vi "wykresy.vi"(8 "error in (no error)":errorcluster, 10 "x*y":dbl[](array[numeric]), 11 "wyjœcie":T1={"Runer's Data"={"Name"="", "Age"=0}, "HR Max"=0, "Raw Data"={"Time"=[], "Bpm"=[]}, "% HR MAX "=[], "HR Zones "=[], "no of points"=[], "Heart Rate Zone No 2"=[], "History"=[["training number", "HR Max value", "HR Mean value"], ["", "", ""]], "number history"=0}) -> (0 "error in (no error) 2":errorcluster, 3 "wyjœcie 2":T1={"Runer's Data"={"Name"="", "Age"=0}, "HR Max"=0, "Raw Data"={"Time"=[], "Bpm"=[]}, "% HR MAX "=[], "HR Zones "=[], "no of points"=[], "Heart Rate Zone No 2"=[], "History"=[["training number", "HR Max value", "HR Mean value"], ["", "", ""]], "number history"=0})   [LabVIEW 2024]
uses:
  zad_3-labview/klaster 4.ctl
  zad_3-labview/klaster.ctl
  zad_3-labview/klaster 2.ctl
panel:
  out "String 2":string
  out "String":string
  out "BPM":cluster{"Time":timestamp[], "Bpm":i32[]}(graph)
  in  "File Path":path
  in  "Button":bool
  out "HEART RATE ZONES":string[][](array[string])
  out "XY Graph":T4(graph)
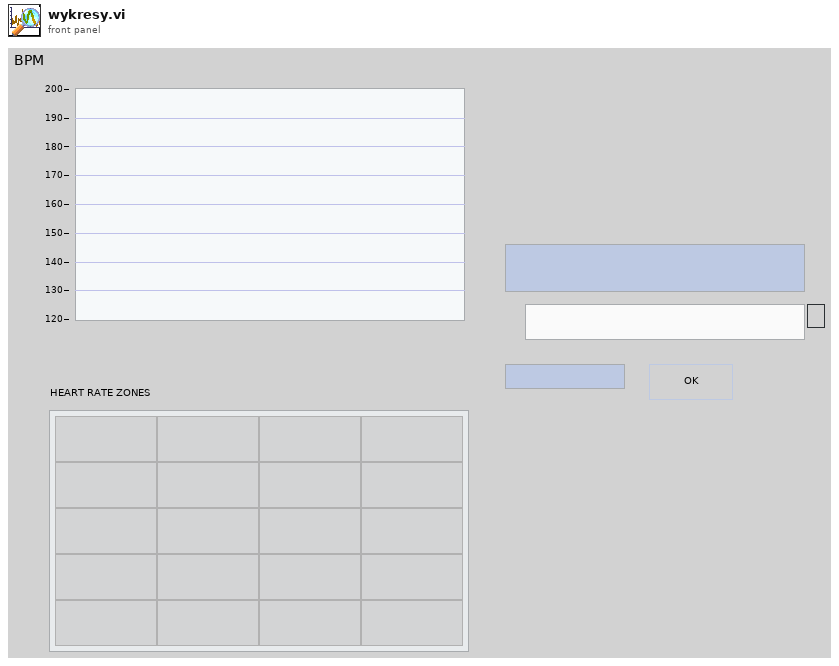
[diagram p1: front panel]
types:
  T1 = typedef "klaster 4.ctl" = cluster{"Runer's Data":T2, "HR Max":i32, "Raw Data":T3, "% HR MAX ":dbl[], "HR Zones ":string[][], "no of points":dbl[], "Heart Rate Zone No 2":i32[], "History":string[][], "number history":i32}
  T2 = typedef "klaster.ctl" = cluster{"Name":string, "Age":i32}
  T3 = typedef "klaster 2.ctl" = cluster{"Time":timestamp[], "Bpm":i32[]}
  T4 = cluster{" Total time in Zone (%) ":dbl[], "Heart Rate Zone":i32[]}
  T5 = cluster{"x*y":dbl[], "Heart Rate Zone No 2":i32[]}
  T6 = typedef "LVCursorListTypeDef.ctl" = cluster{"Name":string, "Color":u32, "Style":u8, "Point Style":u8, "Name Visible":bool, "Allow Drag":bool, "Cursor Mode":u32, "Plot":i32, "Index":i32, "Position":cluster{"X":dbl, "Y":dbl}, "X Scale":u32, "Y Scale":u32, "Watch Plots":i32[], "Watch All Plots":bool, "Plot Area":i32, "Label Offset":cluster{"X":dbl, "Y":dbl}}[]
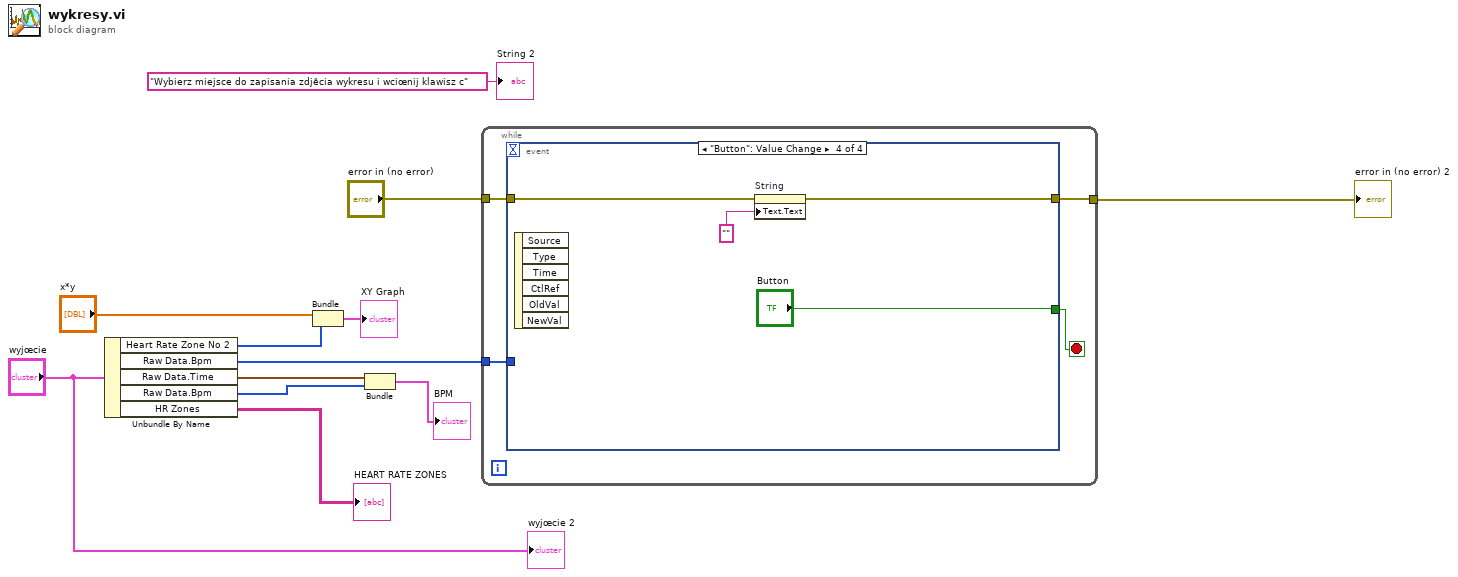
[diagram p0: block diagram]
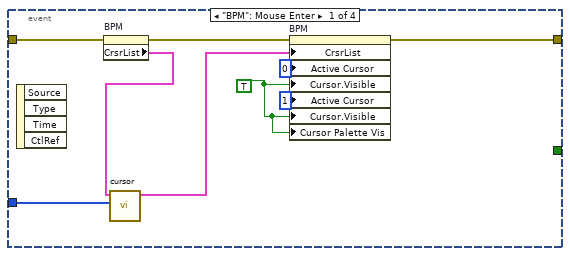
[diagram p2: hidden frame]
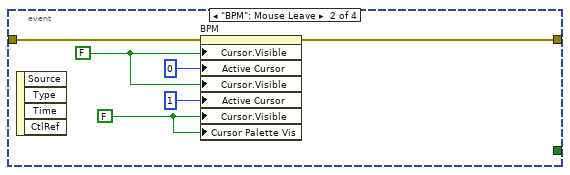
[diagram p3: hidden frame]
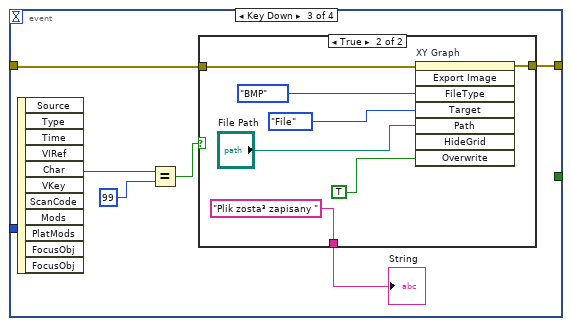
[diagram p4: hidden frame]
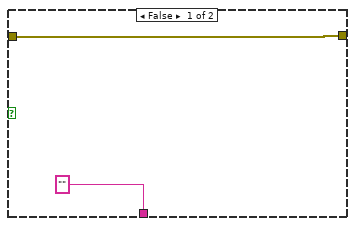
[diagram p5: hidden frame]
diagram:
  n1 = Unbundle By Name("wyjœcie") -> ("Heart Rate Zone No 2"=w7:i32[], "Raw Data.Bpm"=w6:i32[], "Raw Data.Time"=w4:timestamp[], "Raw Data.Bpm"=w2:i32[], "HR Zones"=→"HEART RATE ZONES":string[][])
  n2 = Bundle("x*y"="x*y", "Heart Rate Zone No 2"=w7) -> (→"XY Graph":T5)  [unwired: 1 in]
  n3 = Bundle("Time"=w4, "Bpm"=w2) -> (→"BPM":cluster{"Time":timestamp[], "Bpm":i32[]})  [unwired: 1 in]
  n4 = while {
    tunnel: w6 -> [w13]
    tunnel: [w15] -> w8
    tunnel: "error in (no error)" -> [w14]
    stop <- w16 stop-if-true
    n5 = event shown="[3] \"Button\": Value Change" {
      selector: _ -> [_ _ _ _]
      dyn-events: _ -> [_ _ _ _]
      timeout: _ -> [_ _ _ _]
      tunnel: [_ _ _ "Button"] -> w16
      tunnel: [w23 w28 w37 w47] -> w15
      tunnel: w14 -> [w25 w29 w36 w48]
      tunnel: w13 -> [w22 _ _ _]
      event "BPM": Mouse Enter {
        w19 = TRUE
        n6 = event-data() -> ()  [unwired: 1 in, 4 out]
        n7 = property on="BPM" class="XYGraph (strict)"(error in=w25) -> (error out=w24:errorcluster, "CrsrList"=w18:T6)  [unwired: 1 in, 1 out]
        n8 = call "cursor.vi"("Bpm"=w22, "CrsrList in"=w18) -> ("CrsrList out"=w17:T6)  [unwired: 9 in]
        n9 = property on="BPM" class="XYGraph (strict)"(error in=w24, "CrsrList"=w17, "Active Cursor"=u32 0, "Cursor.Visible"=w19, "Active Cursor"=u32 1, "Cursor.Visible"=w19, "Cursor Palette Vis"=w19) -> (error out=w23:errorcluster)  [unwired: 1 in, 1 out]
      }
      event "BPM": Mouse Leave {
        w26 = FALSE ("Cursor.Visible")
        w27 = FALSE ("Cursor.Visible")
        n10 = event-data() -> ()  [unwired: 1 in, 4 out]
        n11 = property on="BPM" class="XYGraph (strict)"(error in=w29, "Cursor.Visible"=w27, "Active Cursor"=u32 0, "Cursor.Visible"=w27, "Active Cursor"=u32 1, "Cursor.Visible"=w26, "Cursor Palette Vis"=w26) -> (error out=w28:errorcluster)  [unwired: 1 in, 1 out]
      }
      event Key Down {
        n12 = event-data() -> ("Char"=w35:i16)  [unwired: 1 in, 10 out]
        n13 = Equal?(x=w35, y=i16 99) -> (x = y?=w33:bool)
        n14 = case shown="True" w33 {
          tunnel: [w39 w43] -> w37
          tunnel: w36 -> [w39 w42]
          tunnel: ["" ("String") "Plik zosta³ zapisany " ("String")] -> w32
          frame False {
          }
          frame True {
            n15 = invoke on="XY Graph" class="XYGraph (strict)" method="Export Image"(error in=w42, "FileType"=enum32{"BMP", "EPS", "EMF", "PICT"}."BMP" ("File Type"), "Target"=enum32{"File", "Clipboard"}."File", "Path"="File Path", "Overwrite"=TRUE ("Always Overwrite")) -> (error out=w43:errorcluster)  [unwired: 3 in, 7 out]
          }
        }
        "String" <- w32
      }
      event "Button": Value Change {
        n16 = event-data() -> ()  [unwired: 1 in, 6 out]
        n17 = property on="String" class="Str"(error in=w48, "Text.Text"="") -> (error out=w47:errorcluster)  [unwired: 1 in, 1 out]
      }
    }
  }
  "error in (no error) 2" <- w8
  "String 2" <- "Wybierz miejsce do zapisania zdjêcia wykresu i wciœnij klawisz c" ("String 2")
  "wyjœcie 2" <- "wyjœcie"
